vi "Cents2DollarStringSubVI.vi"(11 "Cents":dbl) -> (3 "String":string)   [LabVIEW 2019]
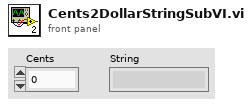
[diagram p1: front panel]
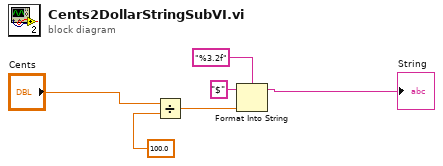
[diagram p0: block diagram]
diagram:
  n1 = Divide(x="Cents", y=100.0) -> (x/y=w3:dbl)
  n2 = Format Into String(format string="%3.2f", initial string="$", w3) -> (resulting string=→"String":string)  [unwired: 1 in, 1 out]
